vi "replace stump vi with user vi.vi"(8 "error in (no error)":errorcluster, 11 "VI in":refnum<vi>) -> (0 "error out":errorcluster, 2 "subvi reference out":refnum<vi>)   [LabVIEW 2013]
uses:
  <vilib>/Utility/traverseref.llb/TRef TravTarget.ctl
  <vilib>/Utility/traverseref.llb/VI Scripting - Traverse.lvlib
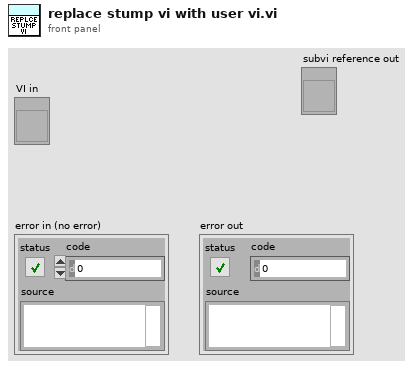
[diagram p1: front panel]
types:
  T1 = typedef "TRef TravTarget.ctl" = enum16{"FP", "BD", "Other"}
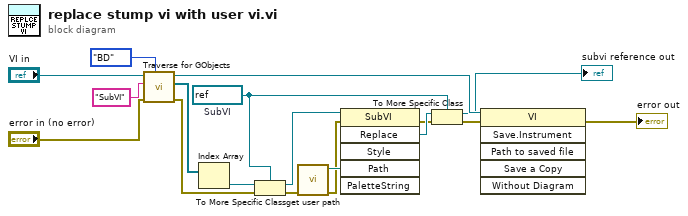
[diagram p0: block diagram]
diagram:
  w6 = refnum<vi> refnum  # SubVI
  n1 = call <vilib>:"Traverse for GObjects.vi"("Traverse Target"=TRef_TravTarget."BD", "error in (no error)"="error in (no error)", "Class Name"="SubVI", "VI Refnum"="VI in") -> ("error out"=w18:errorcluster, "References"=w15:refnum<vi>[], "dup VI Refnum"=w7:refnum<vi>)  [unwired: 4 in, 1 out]
  n2 = Index Array(array=w15) -> (element=w16:refnum<vi>)  [unwired: 1 in]
  n3 = To More Specific Class(target class=w6, reference=w16, error in=w18) -> (specific class reference=w17:refnum<vi>, error out=w9:errorcluster)
  n4 = call "get user path.vi"("error in"=w9) -> ("error out"=w8:errorcluster, "Path"=w10:path)  [unwired: 9 in]
  n5 = invoke class="SubVI" method="Replace"(reference=w17, error in=w8, "Path"=w10) -> (error out=w3:errorcluster, "Replace"=w5:refnum<vi>)  [unwired: 3 in, 4 out]
  n6 = To More Specific Class(target class=w6, reference=w5, error in=w3) -> (specific class reference=→"subvi reference out":refnum<vi>, error out=w2:errorcluster)
  n7 = invoke class="VI" method="Save.Instrument"(reference=w7, error in=w2) -> (error out=→"error out":errorcluster)  [unwired: 4 in, 5 out]
